vi "Append Double.vi"(8 "clear":bool, 9 "Input Array":dbl[](array[numeric]), 10 "Input Vale":dbl, 11 "Update":bool=TRUE) -> (3 "Output Array":dbl[](array[numeric]))   [LabVIEW 2014]
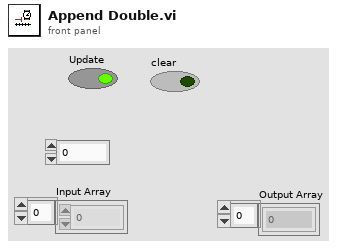
[diagram p1: front panel]
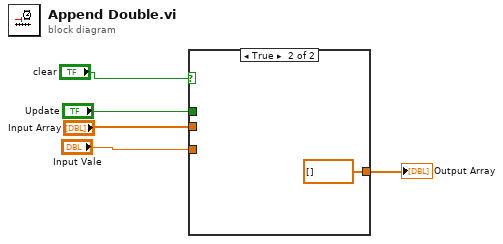
[diagram p0: block diagram]
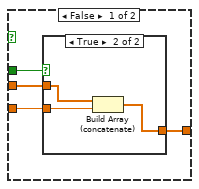
[diagram p2: hidden frame]
diagram:
  n1 = case shown="True" "clear" {
    tunnel: "Input Array" -> [w8 _]
    tunnel: "Update" -> [w9 _]
    tunnel: "Input Vale" -> [w7 _]
    tunnel: [w6 dbl[] [] ("Input Array")] -> w1
    frame False {
      n2 = case shown="True" w9 {
        tunnel: [w10 w13] -> w6
        tunnel: w7 -> [_ w12]
        tunnel: w8 -> [w10 w11]
        frame False {
        }
        frame True {
          n3 = Build Array (concatenate)(w11, w12) -> (w13:dbl[])
        }
      }
    }
    frame True {
    }
  }
  "Output Array" <- w1
